vi "MotionCommExample.vi"   [LabVIEW 2013]
uses:
  TCPCommClass/TCPCommClass.lvclass
  PicoMotorController/Picomoto8742ControllerClass.lvclass
  PicoMotor8472Comm/PicoMotor8742Comm.lvclass
  PicoMotor8742Axis/Picomotor8742Axis.lvclass
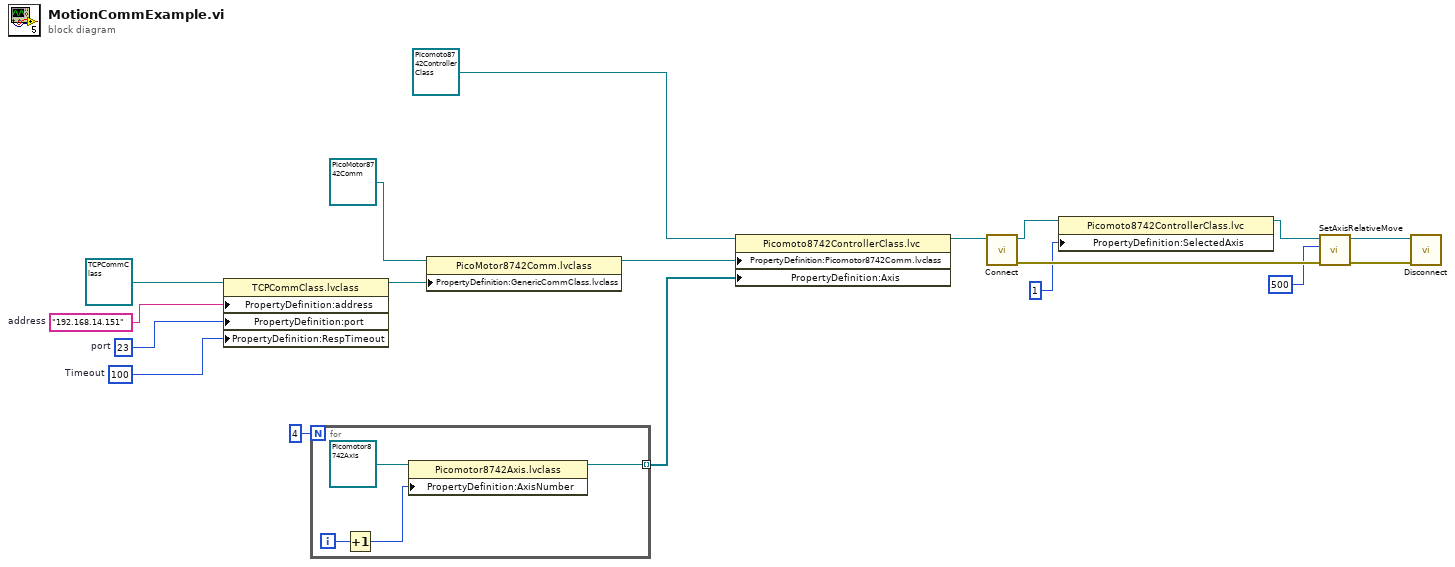
[diagram p0: block diagram]
diagram:
  w15 = u16 100  # Timeout
  w16 = u16 23  # port
  w17 = "192.168.14.151"  # address
  n1 = property class="TCPCommClass.lvclass"(reference=refnum<class "TCPCommClass.lvclass"> refnum ("Picomotor8742Comm in"), "PropertyDefinition:address"=w17, "PropertyDefinition:port"=w16, "PropertyDefinition:RespTimeout"=w15) -> (reference out=w11:refnum<class "TCPCommClass.lvclass">)  [unwired: 1 in, 1 out]
  n2 = for {
    N: 4 -> [_]
    tunnel: [w19] -> w14 mode=indexing
    i -> [w21]
    n3 = Increment(x=w21) -> (x+1=w20:i32)
    n4 = property class="Picomotor8742Axis.lvclass"(reference=refnum<class "Picomotor8742Axis.lvclass"> refnum ("Picomotor8742Axis.lvclass"), "PropertyDefinition:AxisNumber"=w20) -> (reference out=w19:refnum<class "Picomotor8742Axis.lvclass">)  [unwired: 1 in, 1 out]
  }
  n5 = property class="PicoMotor8742Comm.lvclass"(reference=refnum<class "PicoMotor8742Comm.lvclass"> refnum ("PicoMotor8742Comm.lvclass"), "PropertyDefinition:GenericCommClass.lvclass"=w11) -> (reference out=w9:refnum<class "PicoMotor8742Comm.lvclass">)  [unwired: 1 in, 1 out]
  n6 = property class="Picomoto8742ControllerClass.lvc"(reference=refnum<class "Picomoto8742ControllerClass.lvclass"> refnum ("Picomoto8742ControllerClass.lvclass"), "PropertyDefinition:Picomotor8742Comm.lvclass"=w9, "PropertyDefinition:Axis"=w14) -> (reference out=w8:refnum<class "Picomoto8742ControllerClass.lvclass">)  [unwired: 1 in, 1 out]
  n7 = call-dynamic "Connect.vi"("Picomoto8742ControllerClass in"=w8) -> ("error out"=w7:errorcluster, "Picomoto8742ControllerClass out"=w4:refnum<class "Picomoto8742ControllerClass.lvclass">)  [unwired: 9 in]
  n8 = property class="Picomoto8742ControllerClass.lvc"(reference=w4, "PropertyDefinition:SelectedAxis"=u32 1 ("SelectedAxis")) -> (reference out=w3:refnum<class "Picomoto8742ControllerClass.lvclass">)  [unwired: 1 in, 1 out]
  n9 = call-dynamic "SetAxisRelativeMove.vi"("error in (no error)"=w7, "RelativeMovement"=500 ("Acceleration"), "Picomoto8742ControllerClass in"=w3) -> ("error out"=w6:errorcluster, "Picomoto8742ControllerClass out"=w5:refnum<class "Picomoto8742ControllerClass.lvclass">)  [unwired: 7 in]
  n10 = call-dynamic "Disconnect.vi"("error in (no error)"=w6, "Picomoto8742ControllerClass in"=w5) -> ()  [unwired: 8 in, 2 out]
